vi "Hex String To Decimal String.vi"(8 "String":string) -> (0 "Hex String":string)   [LabVIEW 2020]
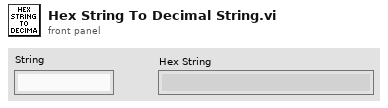
[diagram p1: front panel]
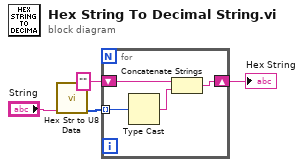
[diagram p0: block diagram]
diagram:
  n1 = call "Hex Str to U8 Data.vi"("HEX String (0-9,A-F)"="String") -> ("u8 Data[]"=w3:u8[])  [unwired: 10 in]
  n2 = for {
    tunnel: w3 -> [w8] mode=indexing
    shift-right: [w5] -> w1
    shift-left: "" -> [w7]
    n3 = Type Cast(x=w8) -> (*(type *) &x=w6:string)  [unwired: 1 in]
    n4 = Concatenate Strings(w7, w6) -> (w5:string)
  }
  "Hex String" <- w1
